vi "Settings Dialog.vi"(8 "error in (no error)":errorcluster, 11 "User Specified Data in":T1={"Hardware Configuration"={"Signal Channel"="", "Response Channel"="", "Trigger Channel"="", "Number of acquisitions"=0.0}, "Analysis Configuration"={"Statistics"=TRUE}, "Signal Type"=enum."Single Chirp", "New Data Behavior"=enum."Replace", "Signal Configuration"={"Chirp Amplitude"=0.1, "I/O Limit"=10.0, "Sample Rate"=1000000.0, "Chirp Duration (s)"=10000000.0, "Upper Frequency"=0.0, "Lower Frequency"=0.0, "Windowing"=enum."None"}}) -> (0 "error out":errorcluster, 2 "UI Refresh Needed?":bool, 3 "User specified data out":T1={"Hardware Configuration"={"Signal Channel"="", "Response Channel"="", "Trigger Channel"="", "Number of acquisitions"=0.0}, "Analysis Configuration"={"Statistics"=TRUE}, "Signal Type"=enum."Single Chirp", "New Data Behavior"=enum."Replace", "Signal Configuration"={"Chirp Amplitude"=0.1, "I/O Limit"=10.0, "Sample Rate"=1000000.0, "Chirp Duration (s)"=10000000.0, "Upper Frequency"=0.0, "Lower Frequency"=0.0, "Windowing"=enum."None"}})   [LabVIEW 2017]
doc: "Dialog for selecting user specified settings."
uses:
  controls/User Specified Data.ctl
  controls/HW Configuration.ctl
  controls/Analysis Configuration.ctl
  controls/New Data Behavior.ctl
  controls/Signal Configuration.ctl
panel:
  in  "No. of Acquisitions":dbl=1.0
  in  "Chirp Amplitude (V)":dbl=10.0
  in  "Input Voltage Limit (V)":dbl=10.0
  in  "Chirp Windowing":u16(ring) items=["None", "Exponential", "Flat top", "Hamming", "Hanning", "Kaiser-Bessel", "Rectangular"]
  in  "Signal Type":u16(ring) items=["Single Chirp", "From Excel"]
  in  "Response Channel":tag="PXI1Slot7/ai0"
  in  "Signal Channel":tag="PXI1Slot7/ao0"
  in  "Trigger Channel":tag="/PXI1Slot7/PFI1"
  in  "Lower Freq. (Hz)":dbl=-10.0
  in  "Upper Freq. (Hz)":dbl=10.0
  in  "Chirp Duration (s)":dbl=1000.0
  in  "Sample Rate (S/s)":dbl=10000.0
  in  "New Data Behavior":u16(ring) items=["Replace", "Overlay", "Append"]
  in  "Cancel Button":bool
  in  "OK Button":bool
  # "0 to acquire \nuntil falling edge"
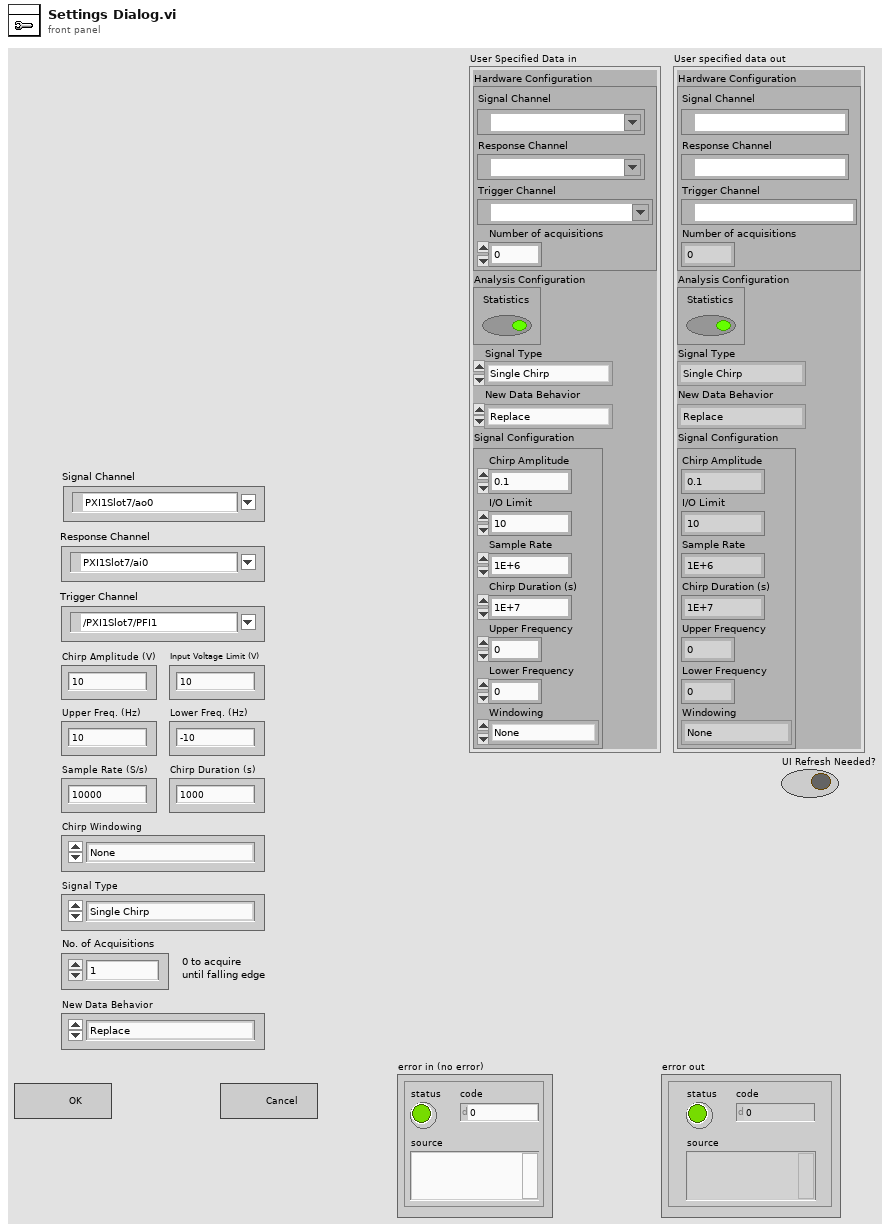
[diagram p1: front panel]
types:
  T1 = typedef "User Specified Data.ctl" = cluster{"Hardware Configuration":T2, "Analysis Configuration":T3, "Signal Type":enum16{"Single Chirp", "From Excel"}, "New Data Behavior":T4, "Signal Configuration":T5}
  T2 = typedef "HW Configuration.ctl" = cluster{"Signal Channel":tag, "Response Channel":tag, "Trigger Channel":tag, "Number of acquisitions":dbl}
  T3 = typedef "Analysis Configuration.ctl" = cluster{"Statistics":bool}
  T4 = typedef "New Data Behavior.ctl" = enum16{"Replace", "Overlay", "Append"}
  T5 = typedef "Signal Configuration.ctl" = cluster{"Chirp Amplitude":dbl, "I/O Limit":dbl, "Sample Rate":dbl, "Chirp Duration (s)":dbl, "Upper Frequency":dbl, "Lower Frequency":dbl, "Windowing":enum16{"None", "Exponential", "Flat top", "Hamming", "Hanning", "Kaiser-Bessel", "Rectangular"}}
  T6 = enum16{"None", "Exponential", "Flat top", "Hamming", "Hanning", "Kaiser-Bessel", "Rectangular"}
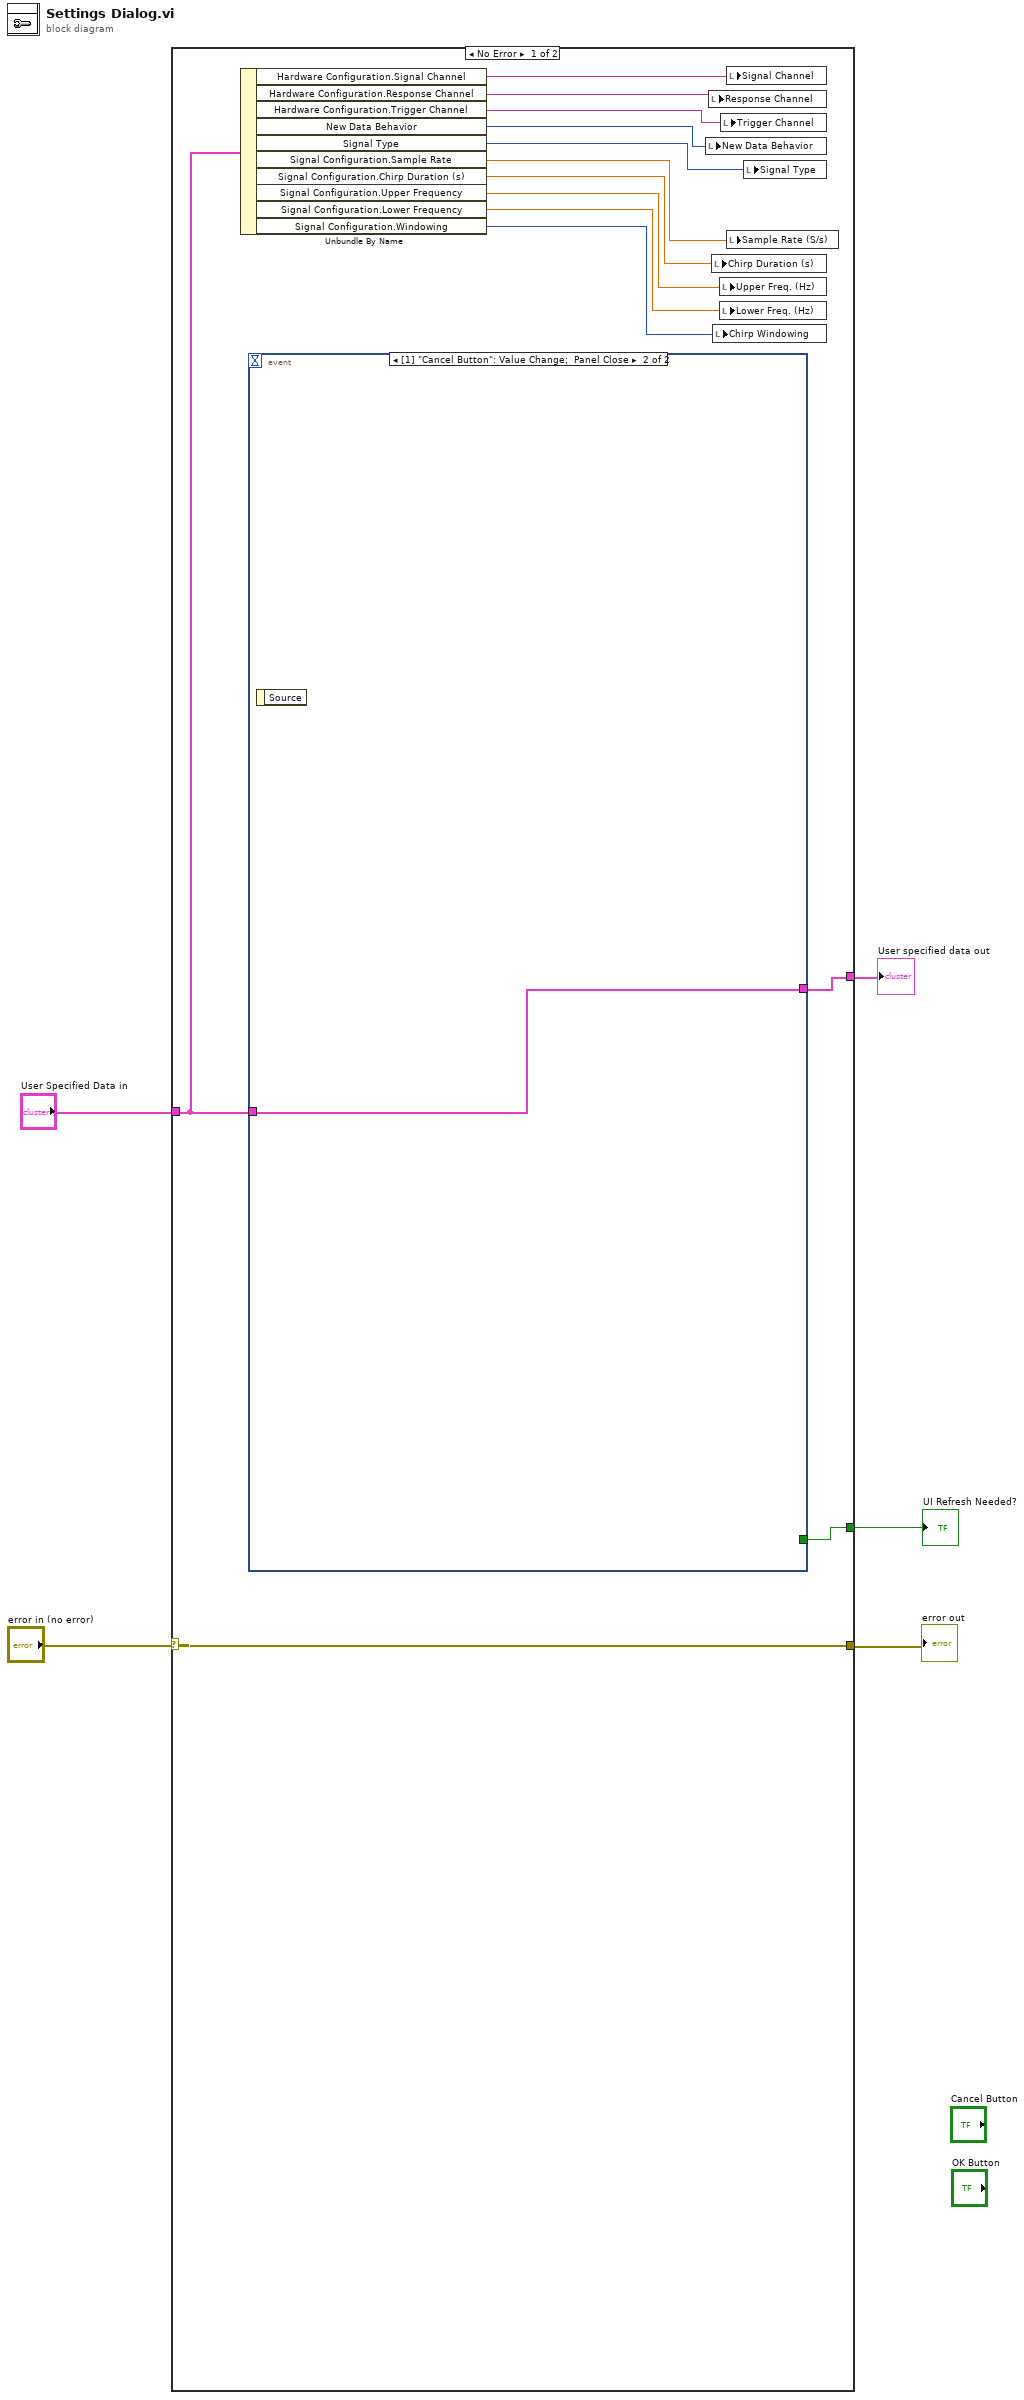
[diagram p0: block diagram]
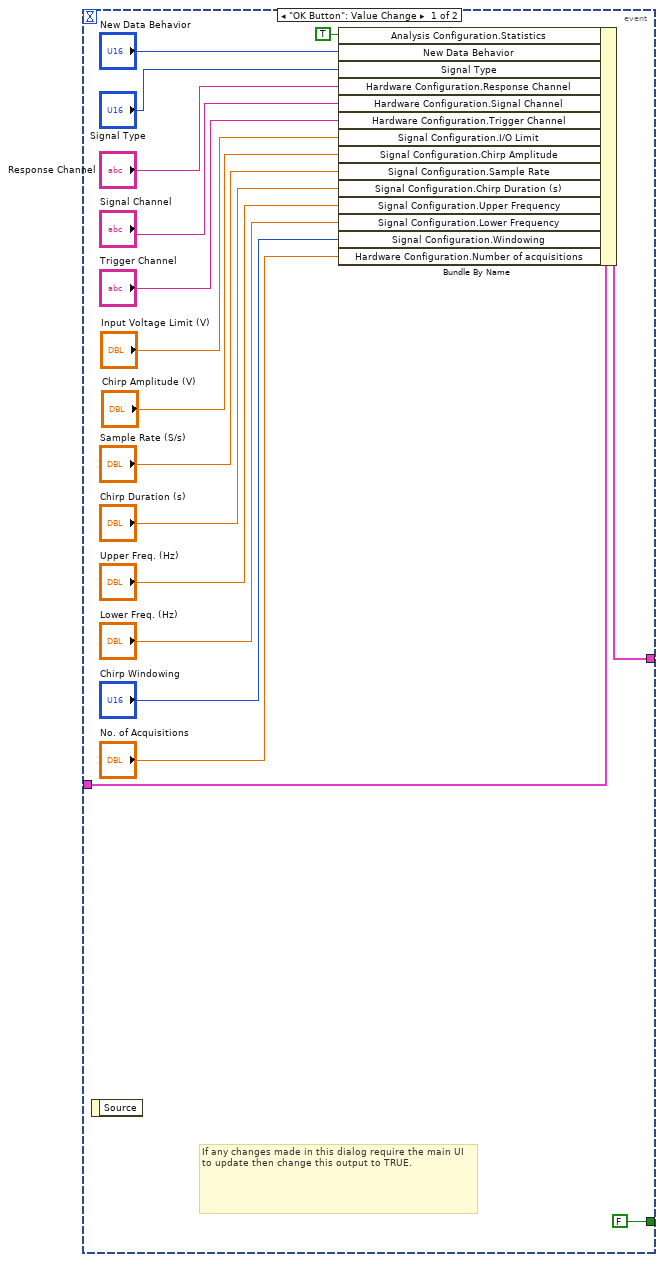
[diagram p2: hidden frame]
diagram:
  n1 = case shown="No Error" "error in (no error)" {
    selector: "error in (no error)" -> [w18 w39]
    tunnel: [w18 w39] -> w4
    tunnel: "User Specified Data in" -> [w14 w38]
    tunnel: [w19 w38] -> w2
    tunnel: [w15 _] -> w1
    frame No Error {
      n2 = Unbundle By Name(w14) -> ("Hardware Configuration.Signal Channel"=w17:tag, "Hardware Configuration.Response Channel"=w16:tag, "Hardware Configuration.Trigger Channel"=w13:tag, "New Data Behavior"=w12:T4, "Signal Type"=w11:enum16{"Single Chirp", "From Excel"}, "Signal Configuration.Sample Rate"=w10:dbl, "Signal Configuration.Chirp Duration (s)"=w9:dbl, "Signal Configuration.Upper Frequency"=w8:dbl, "Signal Configuration.Lower Frequency"=w7:dbl, "Signal Configuration.Windowing"=w6:T6)
      n3 = event shown="[1] \"Cancel Button\": Value Change;  Panel Close" {
        selector: _ -> [_ _]
        dyn-events: _ -> [_ _]
        timeout: _ -> [_ _]
        tunnel: [w36 w37] -> w19
        tunnel: w14 -> [w34 w37]
        tunnel: [FALSE ("UI Refresh Needed?") _] -> w15
        event "OK Button": Value Change {
          # "If any changes made in this dialog require the main UI to update then change this output to TRUE."
          n4 = event-data() -> ()  [unwired: 1 in, 1 out]
          n5 = Bundle By Name(cluster=w34, "Analysis Configuration.Statistics"=TRUE, "New Data Behavior"="New Data Behavior", "Signal Type"="Signal Type", "Hardware Configuration.Response Channel"="Response Channel", "Hardware Configuration.Signal Channel"="Signal Channel", "Hardware Configuration.Trigger Channel"="Trigger Channel", "Signal Configuration.I/O Limit"="Input Voltage Limit (V)", "Signal Configuration.Chirp Amplitude"="Chirp Amplitude (V)", "Signal Configuration.Sample Rate"="Sample Rate (S/s)", "Signal Configuration.Chirp Duration (s)"="Chirp Duration (s)", "Signal Configuration.Upper Frequency"="Upper Freq. (Hz)", "Signal Configuration.Lower Frequency"="Lower Freq. (Hz)", "Signal Configuration.Windowing"="Chirp Windowing", "Hardware Configuration.Number of acquisitions"="No. of Acquisitions") -> (w36:T1)
        }
        event "Cancel Button": Value Change; Panel Close {
          n6 = event-data() -> ()  [unwired: 1 in, 1 out]
        }
      }
      n7 = local write "New Data Behavior"(w12) -> ()
      n8 = local write "Response Channel"(w16) -> ()
      n9 = local write "Chirp Duration (s)"(w9) -> ()
      n10 = local write "Chirp Windowing"(w6) -> ()
      n11 = local write "Upper Freq. (Hz)"(w8) -> ()
      n12 = local write "Lower Freq. (Hz)"(w7) -> ()
      n13 = local write "Trigger Channel"(w13) -> ()
      n14 = local write "Signal Channel"(w17) -> ()
      n15 = local write "Sample Rate (S/s)"(w10) -> ()
      n16 = local write "Signal Type"(w11) -> ()
    }
    frame Error {
    }
  }
  "UI Refresh Needed?" <- w1
  "error out" <- w4
  "User specified data out" <- w2
